vi "pumpSwitch.vi"(8 "error in (no error)":errorcluster, 10 "Sensors":refnum<class "Sensor.lvclass">[](array[class]), 11 "Pump in":refnum<class "Pump.lvclass">) -> (0 "error out":errorcluster, 3 "Pump out":refnum<class "Pump.lvclass">)   [LabVIEW 2017, in "Pump.lvclass"]
uses:
  Pump.lvclass
  Sensor Class/Sensor.lvclass
  Pump.lvclass/Pump.ctl
  Sensor Class/Sensor.lvclass/Sensor.ctl
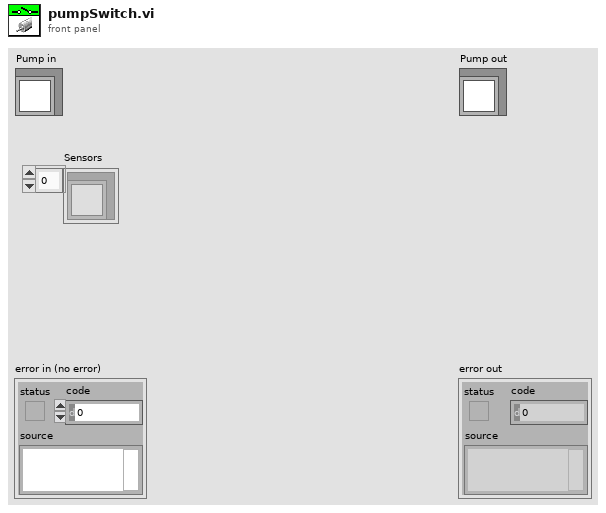
[diagram p1: front panel]
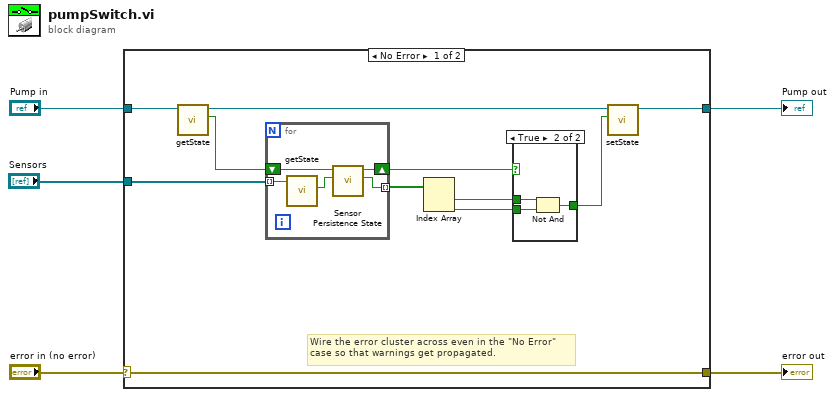
[diagram p0: block diagram]
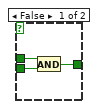
[diagram p2: hidden frame]
diagram:
  n1 = case shown="No Error" "error in (no error)" {
    selector: "error in (no error)" -> [w16 w29]
    tunnel: [w16 w29] -> w4
    tunnel: [w9 w28] -> w2
    tunnel: "Pump in" -> [w11 w28]
    tunnel: "Sensors" -> [w15 _]
    frame No Error {
      # "Wire the error cluster across even in the \"No Error\"\ncase so that warnings get propagated."
      n2 = call "getState.vi"("Pump in"=w11) -> ("state"=w7:bool, "Pump out"=w10:refnum<class "Pump.lvclass">)  [unwired: 8 in, 1 out]
      n3 = for {
        tunnel: w15 -> [w27] mode=indexing
        tunnel: [w25] -> w14 mode=indexing
        shift-right: [w23] -> w6
        shift-left: w7 -> [w24]
        n4 = call "getState.vi"("Sensor in"=w27) -> ("State"=w26:bool)  [unwired: 8 in, 2 out]
        n5 = call "Sensor Persistence State.vi"("Sensor"=w26, "Pump State in"=w24) -> ("Persistent State"=w25:bool, "Pump State out"=w23:bool)  [unwired: 8 in]
      }
      n6 = Index Array(array=w14) -> (element #1=w13:bool, element #2=w12:bool)  [unwired: 2 in]
      n7 = case shown="True" w6 {
        tunnel: w13 -> [w18 w22]
        tunnel: [w19 w21] -> w8
        tunnel: w12 -> [w17 w20]
        frame False {
          n8 = And(x=w18, y=w17) -> (x .and. y?=w19:bool)
        }
        frame True {
          n9 = Not And(1:w20, 2:w22) -> (0:w21:bool)
        }
      }
      n10 = call "setState.vi"("state"=w8, "Pump in"=w10) -> ("Pump out"=w9:refnum<class "Pump.lvclass">)  [unwired: 8 in, 1 out]
    }
    frame Error {
    }
  }
  "error out" <- w4
  "Pump out" <- w2
